vi "Validate_Simulation.vi"() -> ()   [LabVIEW 2020, in "Keysight_34401A-DMM.lvclass"]
uses:
  Keysight_34401A-DMM.lvclass
  <instrlib>/Agilent 34401/Public/Data/Read (Single Point).vi
  <vilib>/MeasurementLink/MeasurementLink Instrument/ISession Factory/Remote Connection Options.ctl
  <vilib>/MeasurementLink/MeasurementLink Instrument/ISession Factory/ISession Factory.lvclass
  <vilib>/MeasurementLink/MeasurementLink Instrument/ISession Factory/Session Initialization Parameters.ctl
  <instrlib>/Agilent 34401/Agilent 34401.lvlib
  <vilib>/MeasurementLink/MeasurementLink Instrument/ISession Factory/Initialize and Close Session Behavior.ctl
panel:
  out "error out":errorcluster
  out "Measurement":dbl
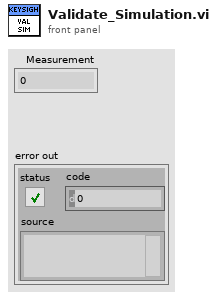
[diagram p1: front panel]
types:
  T1 = typedef "MeasurementLink Instrument.lvlib/ISession Factory.lvclass/Initialize and Close Session Behavior.ctl" = enum16{"Initialize and Close", "Attach and Detach", "Initialize and Detach", "Attach and Close"}
  T2 = typedef "MeasurementLink Instrument.lvlib/ISession Factory.lvclass/Session Initialization Parameters.ctl" = cluster{"resource name":string, "session name":string}
  T3 = typedef "MeasurementLink Instrument.lvlib/ISession Factory.lvclass/Remote Connection Options.ctl" = cluster{"session name":string, "address":string, "port":u32}
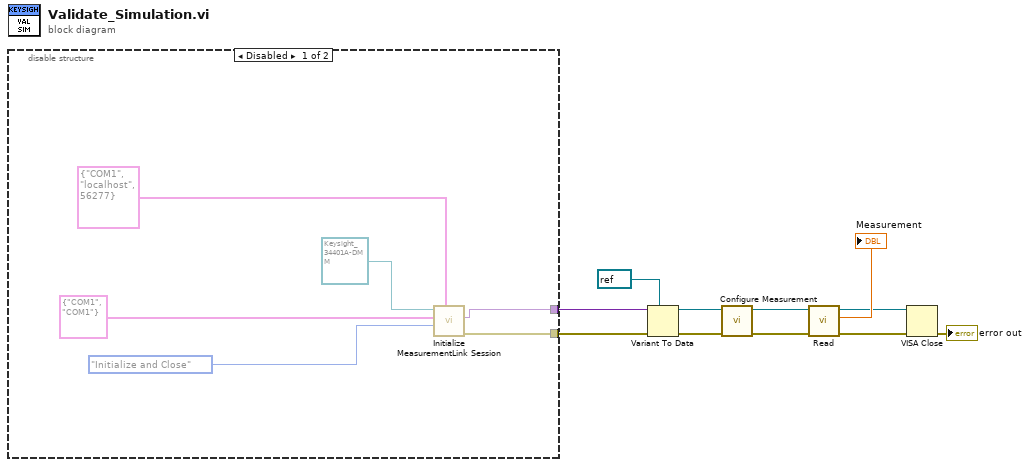
[diagram p0: block diagram]
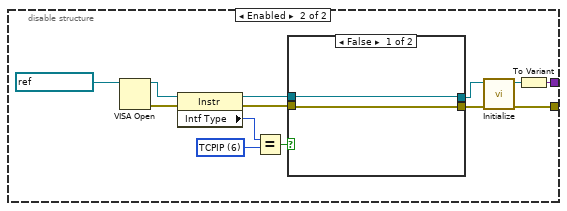
[diagram p2: hidden frame]
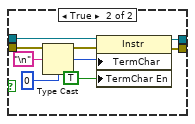
[diagram p3: hidden frame]
diagram:
  n1 = disable-structure shown="Disabled" {
    disable-tunnel: [w15 w29] -> w9
    disable-tunnel: [w14 w27] -> w7
    frame Disabled {
      n2 = call-dynamic "Initialize MeasurementLink Session.vi"("remote connection options"=T3 {"session name"="COM1", "address"="localhost", "port"=56277}, "initialize and close session behavior"=Initialize_and_Close_Session_Behavior."Initialize and Close" ("initialize session behavior"), "session initialization parameters"=T2 {"resource name"="COM1", "session name"="COM1"}, "session factory in"=refnum<class "Keysight_34401A-DMM.lvclass"> refnum) -> ("error out"=w15:errorcluster, "session out"=w14:variant)  [unwired: 5 in, 1 out]
    }
    frame Enabled {
      w20 = u16 6 items=["GPIB"=1, "VXI"=2, "GPIB-VXI"=3, "Serial"=4, "PXI"=5, "TCPIP"=6, "USB"=7, "FireWire"=9] ("Interface Information:Interface Type")
      n3 = VISA Open(VISA resource name=refnum<visa-resource-name> "VISA-TCP") -> (VISA resource name=w22:refnum<visa-resource-name>, error out=w25:errorcluster)  [unwired: 4 in]
      n4 = property class="Instr"(reference=w22, error in=w25) -> (reference out=w21:refnum<visa-resource-name>, error out=w23:errorcluster, "Intf Type"=w19:u16)
      n5 = Equal?(x=w19, y=w20) -> (x = y?=w18:bool)
      n6 = case shown="False" w18 {
        tunnel: [w31 w36] -> w26
        tunnel: [w32 w35] -> w24
        tunnel: w23 -> [w31 w34]
        tunnel: w21 -> [w32 w33]
        frame False {
        }
        frame True {
          n7 = Type Cast(type=u8 0, x="\n" ("Line Feed Constant")) -> (*(type *) &x=w40:u8)
          n8 = property on="Property Node" class="Instr"(reference=w33, error in=w34, "TermChar"=w40, "TermChar En"=TRUE ("Message Based Settings:Termination Character Enable")) -> (reference out=w35:refnum<visa-resource-name>, error out=w36:errorcluster)
        }
      }
      n9 = call <instrlib>:"Initialize.vi"("error in (no error)"=w26, "VISA resource name"=w24) -> ("error out"=w29:errorcluster, "VISA resource name out"=w28:refnum<visa-resource-name>)  [unwired: 8 in]
      n10 = To Variant(anything=w28) -> (Variant=w27:variant)
    }
  }
  n11 = Variant To Data(error in=w9, type=refnum<visa-resource-name> refnum ("VISA resource name"), Variant=w7) -> (data=w2:refnum<visa-resource-name>, error out=w8:errorcluster)
  n12 = call <instrlib>:"Configure Measurement.vi"("error in (no error)"=w8, "VISA resource name"=w2) -> ("error out"=w10:errorcluster, "VISA resource name out"=w11:refnum<visa-resource-name>)  [unwired: 8 in]
  n13 = call-poly <instrlib>:"Read.vi"("error in (no error)"=w10, "VISA resource name"=w11) -> ("error out"=w3:errorcluster, "Measurement"=→"Measurement":dbl, "VISA resource name out"=w4:refnum<visa-resource-name>)  [unwired: 7 in]
  n14 = VISA Close(VISA resource name=w4, error in (no error)=w3) -> (error out=→"error out":errorcluster)
